vi "SafeROI.vi"(2 "ROI in":i32, 3 "Increament":i32) -> (7 "Safe ROI":u32)   [LabVIEW 2020]
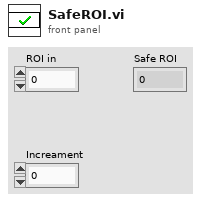
[diagram p1: front panel]
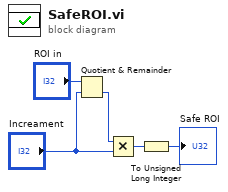
[diagram p0: block diagram]
diagram:
  n1 = Quotient & Remainder(x="ROI in", y="Increament") -> (floor(x/y)=w2:i32)  [unwired: 1 out]
  n2 = Multiply(x=w2, y="Increament") -> (x*y=w4:i32)
  n3 = To Unsigned Long Integer(number=w4) -> (unsigned 32bit integer=→"Safe ROI":u32)
